vi "CleanUp.vi"(0 "object in":refnum<class "AD2_SDK.lvclass">, 5 "error in (no error)":errorcluster) -> (14 "object out":refnum<class "AD2_SDK.lvclass">, 19 "error out":errorcluster)   [LabVIEW 2019, in "AD2_SDK.lvclass"]
uses:
  AD2_SDK.lvclass
  AD2_SDK.lvclass/AD2_SDK.ctl
  InstrumentBase_class/AD2_SDK_class/InstrumentBase.lvclass
  Olasdwf/Olasdwf.lvlib
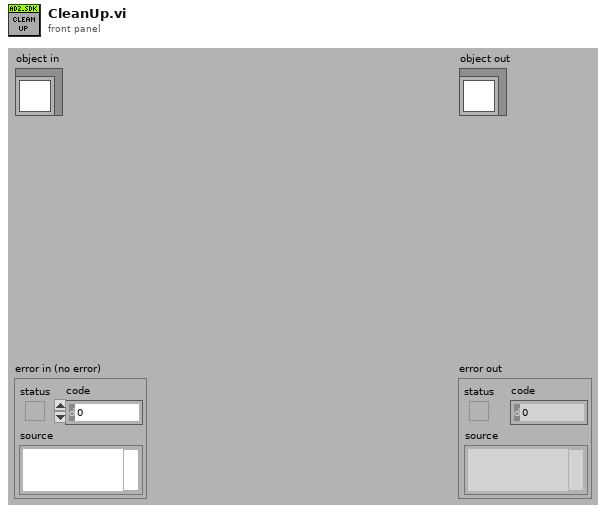
[diagram p1: front panel]
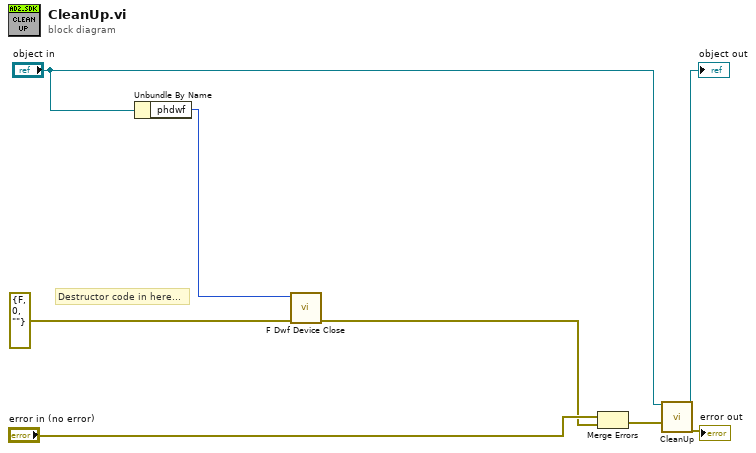
[diagram p0: block diagram]
diagram:
  # "Destructor code in here..."
  n1 = Unbundle By Name("object in") -> ("phdwf"=w7:i32)
  n2 = call "F Dwf Device Close.vi"("error in (no error)"=errorcluster {"status"=FALSE, "code"=0, "source"=""}, "hdwf"=w7) -> ("error out"=w5:errorcluster)  [unwired: 8 in, 1 out]
  n3 = Merge Errors("error in (no error)", w5) -> (w2:errorcluster)
  n4 = call-parent "CleanUp.vi"("object in"="object in", "error in (no error)"=w2) -> ("object out"=→"object out":refnum<class "AD2_SDK.lvclass">, "error out"=→"error out":errorcluster)  [unwired: 16 in]
